vi "BRig_arrTrig_CueLED.vi"() -> (2 "output_CueLED":i32)   [LabVIEW 2014]
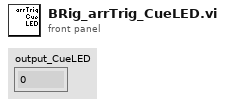
[diagram p1: front panel]
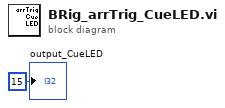
[diagram p0: block diagram]
diagram:
  "output_CueLED" <- 15
